vi "GDSError_SetErrorCustom.vi"(1 "status":bool=TRUE, 3 "source":string, 5 "error in (no error)":errorcluster, 6 "UserDefinedCodes(+5000)":T1) -> (19 "error out":errorcluster)   [LabVIEW 2016]
doc: "You can use this VI to generate errors."
uses:
  <resource>/Framework/Providers/Open_GDS/SubVIs/GOOP_ErrorCodes.ctl
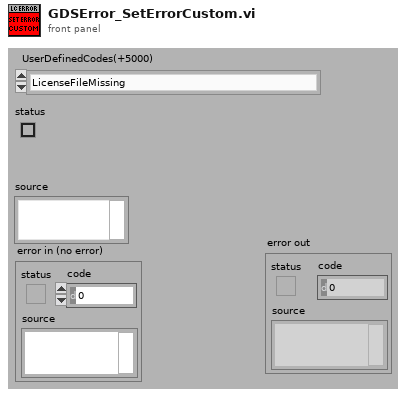
[diagram p1: front panel]
types:
  T1 = typedef "GOOP_ErrorCodes.ctl" = enum16{"LicenseFileMissing", "LicenseFileNotCorrect", "NoProductAccessGranted", "AgreementNoAccepted", "NoValidProviderFound", "LicenseExpired", "LanguageUndefined", "LanguageFileMissing", "LanguageFileChecksumError", "DublicateLanguageTranslation", "LanguageStringIDNotFound", "CommunityLimitReached", "ClassFileLocked", "ClassFileReadOnly", "ProjectNotValid"}
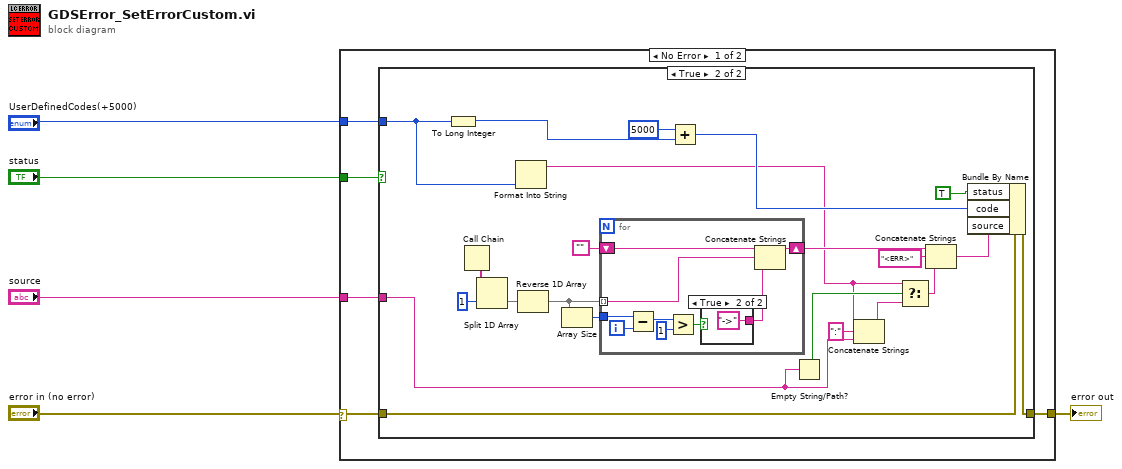
[diagram p0: block diagram]
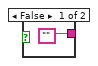
[diagram p3: hidden frame]
diagram:
  n1 = case shown="No Error" "error in (no error)" {
    selector: "error in (no error)" -> [w7 w45]
    tunnel: [w10 w45] -> w5
    tunnel: "status" -> [w9 _]
    tunnel: "source" -> [w8 _]
    tunnel: "UserDefinedCodes(+5000)" -> [w6 _]
    frame No Error {
      n2 = case shown="True" w9 {
        tunnel: w7 -> [w11 w33]
        tunnel: [w11 w32] -> w10
        tunnel: w8 -> [_ w14]
        tunnel: w6 -> [_ w18]
        frame False {
        }
        frame True {
          n3 = To Long Integer(number=w18) -> (32bit integer=w20:i32)
          n4 = Call Chain() -> (call chain=w30:string[])
          n5 = Split 1D Array(array=w30, index=1) -> (second subarray=w28:string[])  [unwired: 1 out]
          n6 = Format Into String(w18) -> (resulting string=w15:string)  [unwired: 3 in, 1 out]
          n7 = Reverse 1D Array(array=w28) -> (reversed array=w22:string[])
          n8 = Array Size(array=w22) -> (size(s)=w27:i32)
          n9 = for {
            shift-right: [w34] -> w25
            shift-left: "" -> [w37]
            tunnel: w22 -> [w35] mode=indexing
            tunnel: w27 -> [w42]
            i -> [w41]
            n10 = Subtract(x=w42, y=w41) -> (x-y=w40:i32)
            n11 = Greater?(x=w40, y=1) -> (0:w38:bool)
            n12 = case shown="True" w38 {
              tunnel: ["" "->"] -> w36
              frame False {
              }
              frame True {
              }
            }
            n13 = Concatenate Strings(w37, w35, w36) -> (w34:string)
          }
          n14 = Add(x=5000, y=w20) -> (x+y=w19:i32)
          n15 = Empty String/Path?(string/path=w14) -> (empty?=w16:bool)
          n16 = Concatenate Strings(w15, ":" ("string"), w14) -> (w13:string)
          n17 = Select(t=w15, s=w16, f=w13) -> (s? t:f=w17:string)
          n18 = Concatenate Strings(w25, "<ERR>" ("Substring"), w17) -> (w26:string)
          n19 = Bundle By Name(cluster=w33, "status"=TRUE ("Bundle Element"), "code"=w19, "source"=w26) -> (w32:errorcluster)
        }
      }
    }
    frame Error {
    }
  }
  "error out" <- w5
